vi "Main Other2.vi"(2 "TSThreadId":u32, 3 "TSThreadCPUAffinity":u32) -> (0 "OutputCPUThreadAffinity":u32[](array[numeric]), 1 "OutputThreadIDArray":u32[](array[numeric]))   [LabVIEW 2012, in "ProjLib.lvlib"]
uses:
  ProjLib.lvlib
panel:
  out "error out":errorcluster
  in  "error in (no error)":errorcluster
  out "CurrentThreadId":u32
  in  "stop":bool
  out "ThreadIdOut2":u32
  out "ThreadIdOut4":u32
  out "ThreadIdOut3":u32
  out "ThreadIdOut1":u32
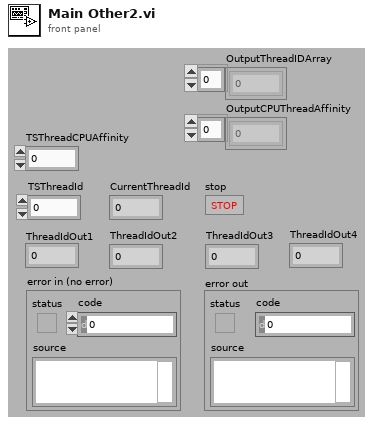
[diagram p1: front panel]
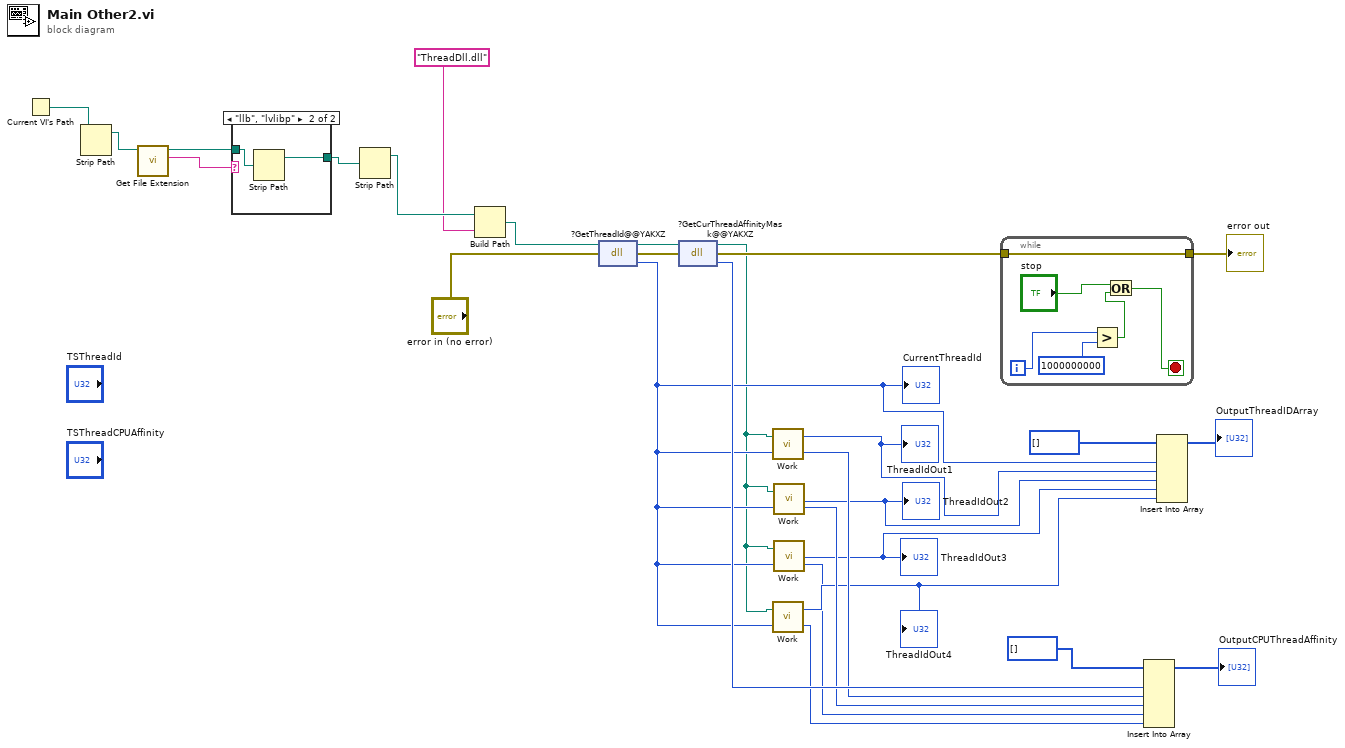
[diagram p0: block diagram]
diagram:
  n1 = Current VI's Path() -> (path=w28:path)
  n2 = Strip Path(path=w28) -> (stripped path=w25:path)  [unwired: 1 out]
  n3 = call "Get File Extension.vi"("file"=w25) -> ("lowercase file extension"=w27:string, "dup file"=w26:path)  [unwired: 7 in, 2 out]
  n4 = case shown="\"llb\", \"lvlibp\"" w27 {
    tunnel: w26 -> [w29 w31]
    tunnel: [w29 w30] -> w24
    frame Default {
    }
    frame "llb", "lvlibp" {
      n5 = Strip Path(path=w31) -> (stripped path=w30:path)  [unwired: 1 out]
    }
  }
  n6 = Strip Path(path=w24) -> (stripped path=w23:path)  [unwired: 1 out]
  n7 = Build Path(base path=w23, name or relative path="ThreadDll.dll") -> (appended path=w20:path)
  n8 = dll-call lib="ThreadDll.dll" fn="?GetThreadId@@YAKXZ"(path in=w20, error in="error in (no error)") -> (path out=w18:path, error out=w19:errorcluster, "return type"=w15:u32)  [unwired: 1 in]
  "CurrentThreadId" <- w15
  n9 = dll-call lib="ThreadDll.dll" fn="?GetCurThreadAffinityMask@@YAKXZ"(path in=w18, error in=w19) -> (path out=w1:path, error out=w17:errorcluster, "return type"=w16:u32)  [unwired: 1 in]
  n10 = call "Work.vi"("ThreadIdIn"=w15, "Dll Path"=w1) -> ("CPUThreadAffinity"=w13:u32, "UsedThreadId"=w14:u32)
  "ThreadIdOut1" <- w14
  n11 = call "Work.vi"("ThreadIdIn"=w15, "Dll Path"=w1) -> ("CPUThreadAffinity"=w7:u32, "UsedThreadId"=w9:u32)
  "ThreadIdOut4" <- w9
  n12 = call "Work.vi"("ThreadIdIn"=w15, "Dll Path"=w1) -> ("CPUThreadAffinity"=w12:u32, "UsedThreadId"=w11:u32)
  "ThreadIdOut2" <- w11
  n13 = call "Work.vi"("ThreadIdIn"=w15, "Dll Path"=w1) -> ("CPUThreadAffinity"=w8:u32, "UsedThreadId"=w10:u32)
  "ThreadIdOut3" <- w10
  n14 = while {
    tunnel: w17 -> [w37]
    tunnel: [w37] -> w6
    i -> [w36]
    stop <- w32 stop-if-true
    n15 = Greater?(x=w36, y=1000000000) -> (0:w34:bool)
    n16 = Or(x="stop", y=w34) -> (x .or. y?=w32:bool)
  }
  "error out" <- w6
  n17 = Insert Into Array(array=u32[] [], new element #1=w16, new element #2=w13, new element #3=w12, new element #4=w8, new element #5=w7) -> (→"OutputCPUThreadAffinity":u32[])  [unwired: 1 in]
  n18 = Insert Into Array(array=u32[] [], new element #1=w15, new element #2=w14, new element #3=w11, new element #4=w10, new element #5=w9) -> (→"OutputThreadIDArray":u32[])  [unwired: 1 in]
